vi "Configure - Load Logo Picture.vi"(7 "hse-config":refnum<class "config-base.lvclass">, 8 "error in (no error)":errorcluster, 11 "Picture Control Ref":refnum<vi>) -> (0 "error out":errorcluster)   [LabVIEW 2022 SP3, in "UI Manager.lvlib"]
doc: "Loads the logo picture as defined in the UI Manager's configuration file into the picture control in <b>Picture Control Ref</b>\n\n____\nHAMPEL SOFTWARE ENGINEERING v2.6.0 (2023-12-19 10:54)"
uses:
  UI Manager.lvlib
  Libraries/hse-libraries/Source/hse-configuration/config-base/config-base.lvclass
  Libraries/hse-libraries/Source/hse-application/hse-application.lvclass/hse-application.ctl
  Libraries/hse-libraries/Source/hse-application/HSE Application not initialized--error.vi
  <vilib>/Utility/error.llb/Clear Errors.vi
  Libraries/hse-libraries/Source/hse-application/hse-application__GetSingleton.vi
  <vilib>/Utility/sysdir.llb/Get System Directory.vi
  <vilib>/Utility/error.llb/Error Cluster From Error Code.vi
  Libraries/hse-libraries/Source/hse-application/hse-application.lvclass
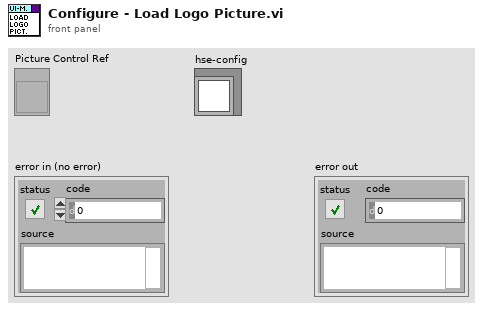
[diagram p1: front panel]
types:
  T1 = typedef "imagedata.ctl" = cluster{"image type":i32, "image depth":i32, "image":u8[], "mask":u8[], "colors":u32[], "Rectangle":cluster{"left":i16, "top":i16, "right":i16, "bottom":i16}}
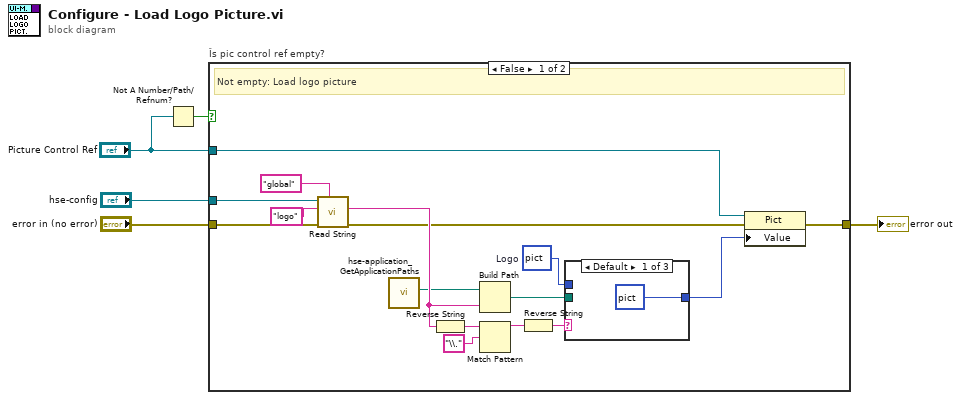
[diagram p0: block diagram]
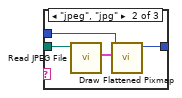
[diagram p2: hidden frame]
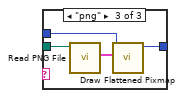
[diagram p3: hidden frame]
diagram:
  n1 = Not A Number/Path/Refnum?(number/path/refnum="Picture Control Ref") -> (NaN/Path/Refnum?=w1:bool)
  n2 = case "Îs pic control ref empty?" shown="False" w1 {
    tunnel: "error in (no error)" -> [w12 w31]
    tunnel: "hse-config" -> [w11 _]
    tunnel: "Picture Control Ref" -> [w10 _]
    tunnel: [w7 w31] -> w3
    frame False {
      w21 = picture data[5B]  # Logo
      # "Not empty: Load logo picture"
      n3 = call-dynamic "Read String.vi"("Section"="global", "error in"=w12, "Key"="logo", "config-base in"=w11) -> ("error out"=w8:errorcluster, "Value"=w20:string)  [unwired: 5 in, 1 out]
      n4 = call "hse-application_GetApplicationPaths.vi"() -> ("Config Directory"=w14:path)  [unwired: 5 in, 6 out]
      n5 = Reverse String(1:w20) -> (0:w15:string)
      n6 = Build Path(base path=w14, name or relative path=w20) -> (appended path=w18:path)
      n7 = Match Pattern(string=w15, regular expression="\\.") -> (before substring=w16:string)  [unwired: 1 in, 3 out]
      n8 = Reverse String(1:w16) -> (0:w17:string)
      n9 = case shown="Default" w17 {
        tunnel: [picture data[5B] ("new picture") w24 w29] -> w9
        tunnel: w18 -> [_ w26 w28]
        tunnel: w21 -> [_ w23 w27]
        frame Default {
        }
        frame "jpeg", "jpg" {
          n10 = call <vilib>:"Read JPEG File.vi"("path to JPEG file"=w26) -> ("image data"=w25:T1)  [unwired: 8 in, 2 out]
          n11 = call <vilib>:"Draw Flattened Pixmap.vi"("image data"=w25, "picture"=w23) -> ("new picture"=w24:picture)  [unwired: 7 in]
        }
        frame "png" {
          n12 = call <vilib>:"Read PNG File.vi"("path to PNG file"=w28) -> ("image data"=w30:T1)  [unwired: 8 in, 2 out]
          n13 = call <vilib>:"Draw Flattened Pixmap.vi"("image data"=w30, "picture"=w27) -> ("new picture"=w29:picture)  [unwired: 7 in]
        }
      }
      n14 = property class="Pict"(reference=w10, error in=w8, "Value"=w9) -> (error out=w7:errorcluster)  [unwired: 1 out]
    }
    frame True {
      # "Empty: Do nothing"
    }
  }
  "error out" <- w3
